vi "rethinkdb_msg_scramsha256.vi"(9 "iteration count":i32, 10 "salt":string, 11 "string":string) -> (3 "sha-256 hash":u32[](array[numeric]) format="%08x")   [LabVIEW 2017]
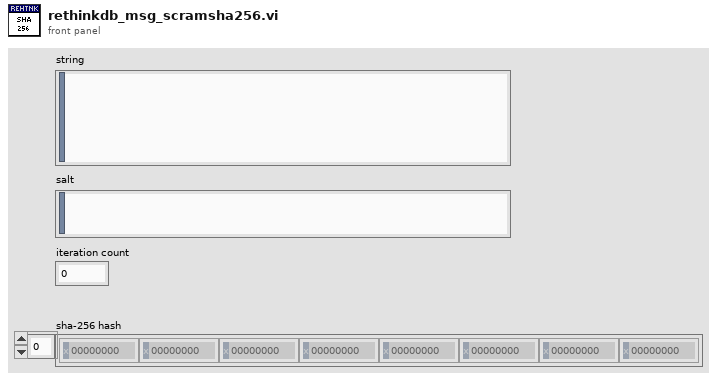
[diagram p1: front panel]
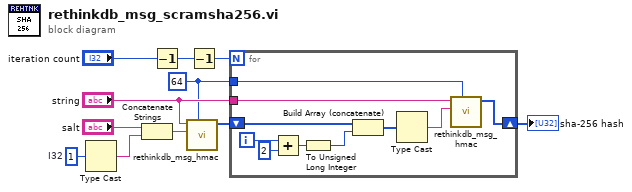
[diagram p0: block diagram]
diagram:
  w8 = 1  # I32
  w4 = 64 ("blocksize (SHA256=64)")
  n1 = Type Cast(x=w8) -> (*(type *) &x=w10:string)  [unwired: 1 in]
  n2 = Concatenate Strings("salt", w10) -> (w6:string)
  n3 = Decrement(x="iteration count") -> (x-1=w2:i32)
  n4 = call "rethinkdb_msg_hmac.vi"("blocksize (SHA256=64)"=w4, "message"=w6, "key"="string") -> ("sha-256 hash"=w5:u32[])  [unwired: 8 in]
  n5 = Decrement(x=w2) -> (x-1=w1:i32)
  n6 = for {
    N: w1 -> [_]
    tunnel: "string" -> [w21]
    shift-right: [w12] -> w3
    shift-left: w5 -> [w18]
    tunnel: w4 -> [w14]
    i -> [w20]
    n7 = Add(x=w20, y=2) -> (x+y=w17:i32)
    n8 = To Unsigned Long Integer(number=w17) -> (unsigned 32bit integer=w16:u32)
    n9 = Build Array (concatenate)(w18, w16) -> (w15:u32[])
    n10 = Type Cast(x=w15) -> (*(type *) &x=w13:string)  [unwired: 1 in]
    n11 = call "rethinkdb_msg_hmac.vi"("blocksize (SHA256=64)"=w14, "message"=w13, "key"=w21) -> ("sha-256 hash"=w12:u32[])  [unwired: 8 in]
  }
  "sha-256 hash" <- w3
